vi "MQTT_PingResp_Read.vi"(8 "error in (no error)":errorcluster, 9 "timeout ms (25000)":i32=25000, 11 "connection ID":refnum<k5>) -> (0 "error out":errorcluster, 2 "ok":bool, 3 "connection ID out":refnum<k5>)   [LabVIEW 2018, in "MQTT_Functions.lvlib"]
uses:
  MQTT_Functions.lvlib
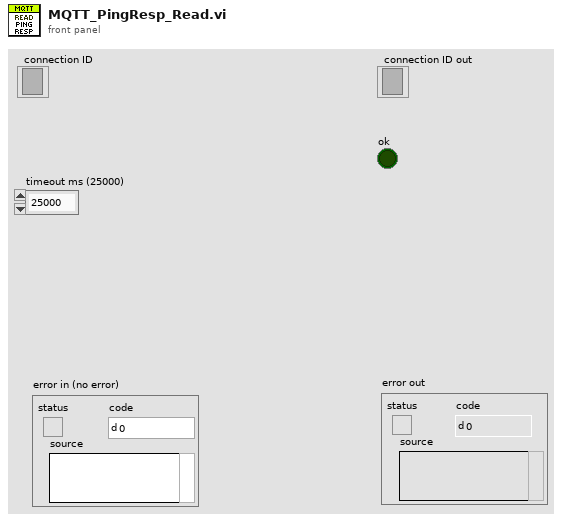
[diagram p1: front panel]
types:
  T1 = typedef "MQTT_Functions.lvlib/MessageType.ctl" = enum32{"Reserved", "CONNECT", "CONNACK", "PUBLISH", "PUBACK", "PUBREC", "PUBREL", "PUBCOMP", "SUBSCRIBE", "SUBACK", "UNSUBSCRIBE", "UNSUBACK", "PINGREQ", "PINGRESP", "DISCONNECT", "Reserved2"}
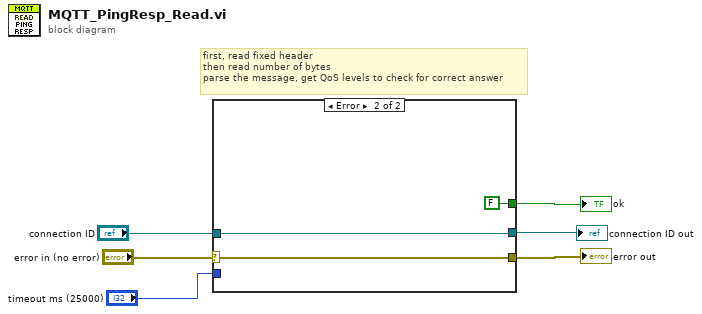
[diagram p0: block diagram]
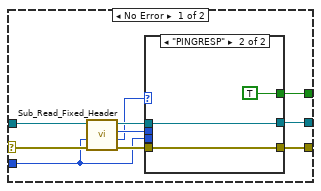
[diagram p2: hidden frame]
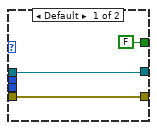
[diagram p3: hidden frame]
diagram:
  # "first, read fixed header\nthen read number of bytes\nparse the message, get QoS levels to check for correct answer"
  n1 = case shown="Error" "error in (no error)" {
    selector: "error in (no error)" -> [w13 w25]
    tunnel: [w12 w25] -> w5
    tunnel: "timeout ms (25000)" -> [w11 _]
    tunnel: "connection ID" -> [w10 w24]
    tunnel: [w9 w24] -> w2
    tunnel: [w7 FALSE] -> w1
    frame No Error {
      n2 = call "Sub_Read_Fixed_Header.vi"("error in (no error)"=w13, "timeout ms (25000)"=w11, "connection ID"=w10) -> ("error out"=w15:errorcluster, "MessageType"=w8:T1, "Remaining Length"=w16:u32, "connection ID out"=w14:refnum<k5>)  [unwired: 2 in, 3 out]
      n3 = case shown="\"PINGRESP\"" w8 {
        tunnel: w16 -> [_ _]
        tunnel: w15 -> [w18 w20]
        tunnel: w14 -> [w19 w22]
        tunnel: [w18 w20] -> w12
        tunnel: w11 -> [_ _]
        tunnel: [w19 w22] -> w9
        tunnel: [FALSE TRUE] -> w7
        frame Default {
        }
        frame "PINGRESP" {
        }
      }
    }
    frame Error {
    }
  }
  "error out" <- w5
  "connection ID out" <- w2
  "ok" <- w1
